vi "Counts Things in the Last Second.vi"(4 "Things to Count":i32) -> (1 "Counts In Last Second":i32)   [LabVIEW 2021]
uses:
  <vilib>/Utility/High Resolution Relative Seconds.vi
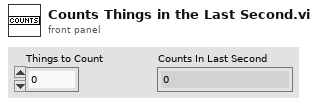
[diagram p1: front panel]
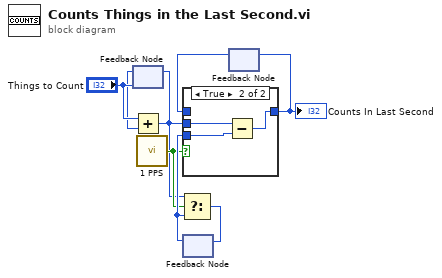
[diagram p0: block diagram]
diagram:
  n1 = feedback #1("Things to Count") -> (w2:i32)
  n2 = Add(x="Things to Count", y=w2) -> (x+y=w1:i32)
  n3 = feedback-in #1(w1) -> ()
  n4 = call "1 PPS.vi"() -> ("1PPS"=w4:bool)  [unwired: 14 in, 1 out]
  n5 = feedback #2() -> (w5:i32)  [unwired: 1 in]
  n6 = Select(t=w1, s=w4, f=w5) -> (s? t:f=w3:i32)
  n7 = feedback-in #2(w3) -> ()
  n8 = feedback #3() -> (w6:i32)  [unwired: 1 in]
  n9 = case shown="True" w4 {
    tunnel: w1 -> [_ w12]
    tunnel: w5 -> [_ w11]
    tunnel: [w9 w10] -> w7
    tunnel: w6 -> [w9 _]
    frame False {
    }
    frame True {
      n10 = Subtract(x=w12, y=w11) -> (x-y=w10:i32)
    }
  }
  "Counts In Last Second" <- w7
  n11 = feedback-in #3(w7) -> ()
